vi "CurrentFunction.vi"(8 "error in":errorcluster, 10 "Function In":string(combo), 11 "Action":enum16{"Set", "Get"}(ring)) -> (0 "error out":errorcluster, 2 "Function Out":string(combo))   [LabVIEW 2016]
doc: "Return the right function when button \"E\" is clicked:\n- Account check\n- Deposit\n- Withdraw"
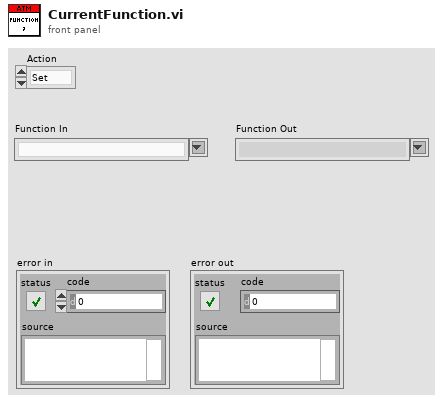
[diagram p1: front panel]
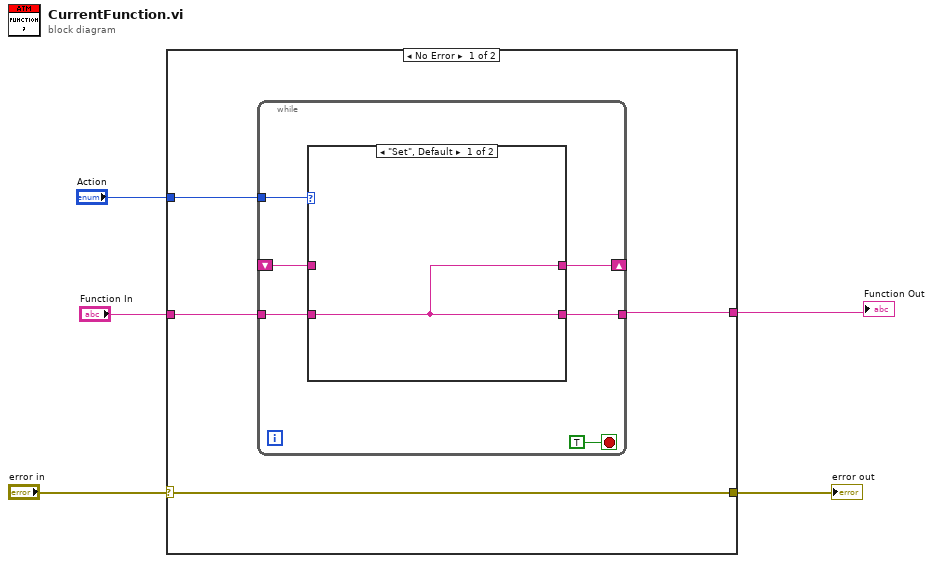
[diagram p0: block diagram]
diagram:
  n1 = case shown="No Error" "error in" {
    selector: "error in" -> [w6 w19]
    tunnel: "Action" -> [w9 _]
    tunnel: "Function In" -> [w8 w18]
    tunnel: [w7 w18] -> w3
    tunnel: [w6 w19] -> w1
    frame No Error {
      n2 = while {
        tunnel: w9 -> [w14]
        tunnel: w8 -> [w12]
        shift-right: [w13] -> _
        shift-left: _ -> [w10]
        tunnel: [w11] -> w7
        stop <- TRUE stop-if-true
        n3 = case shown="\"Set\", Default" w14 {
          tunnel: [w16 w17] -> w13
          tunnel: w12 -> [w16 _]
          tunnel: [w16 w17] -> w11
          tunnel: w10 -> [_ w17]
          frame "Set", Default {
          }
          frame "Get" {
          }
        }
      }
    }
    frame Error {
    }
  }
  "Function Out" <- w3
  "error out" <- w1
